vi "Get position.vi"(8 "error in (no error)":errorcluster, 11 "AlphaStep One in":refnum<class "AlphaStep One.lvclass">) -> (0 "error out":errorcluster, 2 "Voltage (V)":dbl, 3 "AlphaStep One out":refnum<class "AlphaStep One.lvclass">)   [LabVIEW 2018, in "AlphaStep One.lvclass"]
uses:
  AlphaStep One.lvclass
  AlphaStep One.lvclass/AlphaStep One.ctl
  <vilib>/DAQmx/read.llb/DAQmx Read (Analog DBL 1Chan 1Samp).vi
  <vilib>/DAQmx/miscellaneous.llb/DAQmx Fill In Error Info.vi
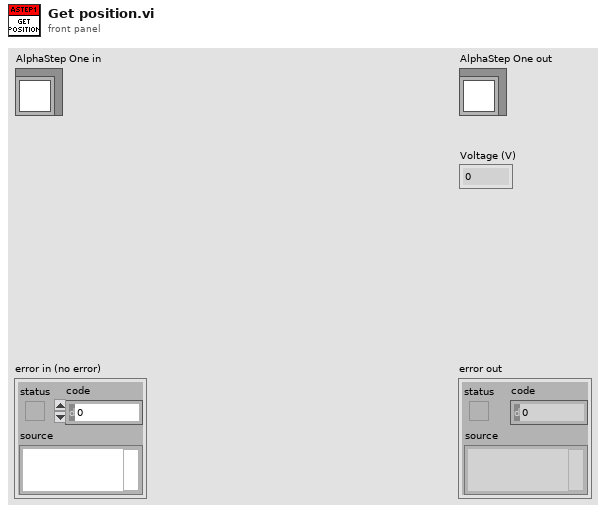
[diagram p1: front panel]
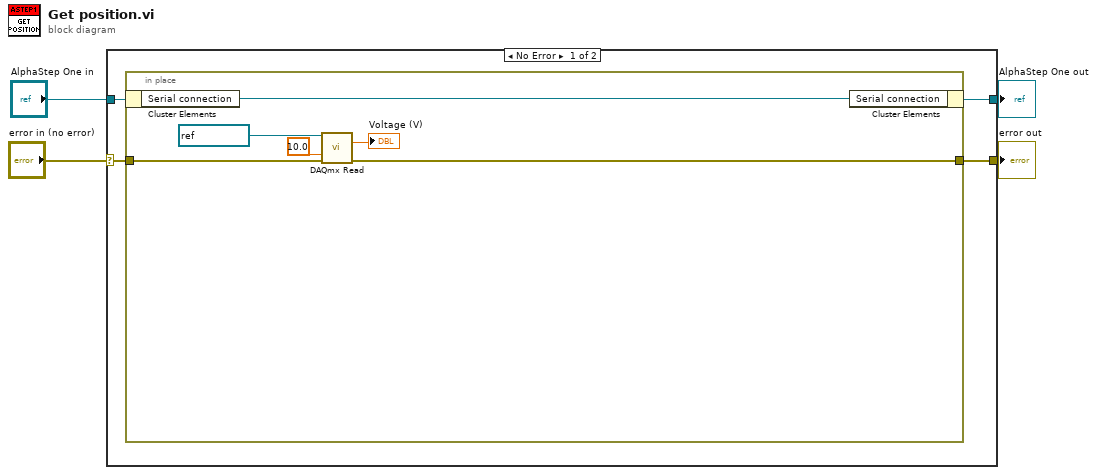
[diagram p0: block diagram]
diagram:
  n1 = case shown="No Error" "error in (no error)" {
    selector: "error in (no error)" -> [w7 w16]
    tunnel: [w6 w16] -> w3
    tunnel: [w5 w15] -> w1
    tunnel: "AlphaStep One in" -> [w8 w15]
    frame No Error {
      n2 = in-place {
        in-place-border: w7 -> [w10]
        in-place-border: [w9] -> w6
        n3 = in-place-cluster #1(w8) -> ("Serial connection"=w14:refnum<class "Serial Device.lvclass">)
        n4 = call-poly <vilib>:"DAQmx Read.vi"("task/channels in"=refnum<k21> "Encoder Voltage" ("DAQmx Global Channel"), "timeout"=10.0, "error in"=w10) -> ("data"=→"Voltage (V)":dbl, "error out"=w9:errorcluster)  [unwired: 10 in, 1 out]
        n5 = in-place-cluster #1("Serial connection"=w14) -> (w5:refnum<class "AlphaStep One.lvclass">)
      }
    }
    frame Error {
    }
  }
  "error out" <- w3
  "AlphaStep One out" <- w1
